vi "Get Component Thickness Temp.vi"() -> (1 "Component Thickness out":dbl)   [LabVIEW 2021, in "Test VIs.lvclass"]
uses:
  Test VIs/Test VIs.lvclass
panel:
  in  "submit":bool
  in  "Enter Component Thickness":dbl
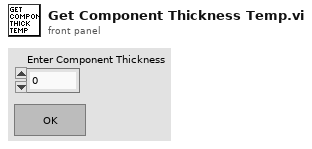
[diagram p1: front panel]
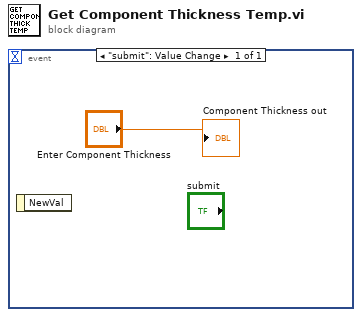
[diagram p0: block diagram]
diagram:
  n1 = event shown="[0] \"submit\": Value Change" {
    selector: _ -> [_]
    dyn-events: _ -> [_]
    timeout: _ -> [_]
    event "submit": Value Change {
      n2 = event-data() -> ()  [unwired: 1 in, 1 out]
      "Component Thickness out" <- "Enter Component Thickness"
    }
  }
